vi "Set New Frame Name.vi"(8 "error in (no error)":errorcluster, 10 "reference in":refnum<vi>, 11 "Getter Generator in":refnum<class "Getter Generator.lvclass">) -> (0 "error out":errorcluster, 2 "reference out":refnum<vi>, 3 "Getter Generator out":refnum<class "Getter Generator.lvclass">)   [LabVIEW 2020, in "Method Generation.lvlib" / "Getter Generator.lvclass"]
uses:
  Getter Generator.lvclass
  Getter Generator.lvclass/Getter Generator.ctl
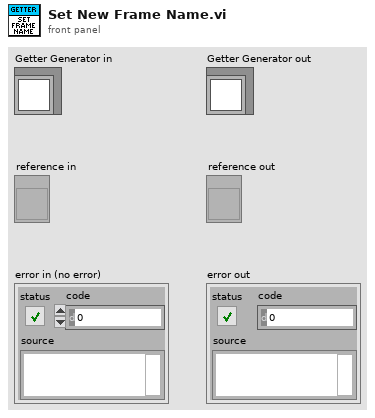
[diagram p1: front panel]
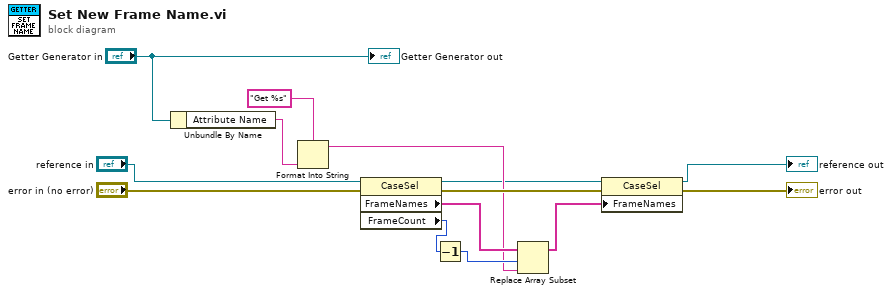
[diagram p0: block diagram]
diagram:
  n1 = Unbundle By Name("Getter Generator in") -> ("Attribute Name"=w9:string)
  n2 = Format Into String(format string="Get %s", w9) -> (resulting string=w5:string)  [unwired: 2 in, 1 out]
  n3 = property class="CaseSel"(reference="reference in", error in="error in (no error)") -> (reference out=w3:refnum<vi>, error out=w14:errorcluster, "FrameNames"=w8:string[], "FrameCount"=w7:i32)
  n4 = Decrement(x=w7) -> (x-1=w6:i32)
  n5 = Replace Array Subset(array=w8, new element=w5, index=w6) -> (w1:string[])
  n6 = property class="CaseSel"(reference=w3, error in=w14, "FrameNames"=w1) -> (reference out=→"reference out":refnum<vi>, error out=→"error out":errorcluster)
  "Getter Generator out" <- "Getter Generator in"
